vi "Write Error code.vi"(8 "error in (no error)":errorcluster, 10 "Error code":string, 11 "data_loader in":refnum<class "data_loader.lvclass">) -> (0 "error out":errorcluster, 3 "data_loader out":refnum<class "data_loader.lvclass">)   [LabVIEW 2017, in "data_loader.lvclass"]
uses:
  data_loader.lvclass
  data_loader.lvclass/data_loader.ctl
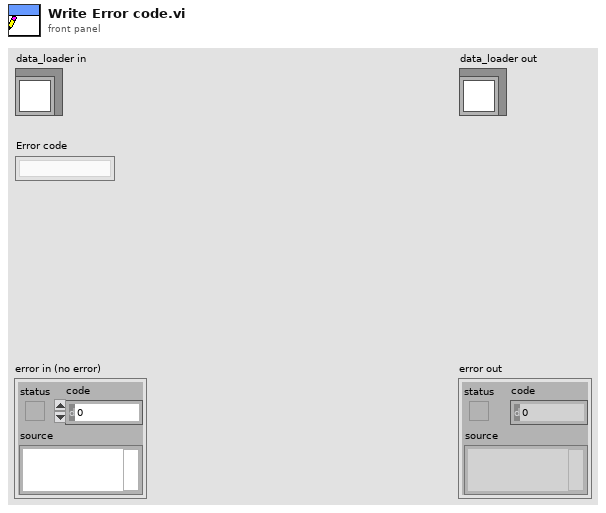
[diagram p1: front panel]
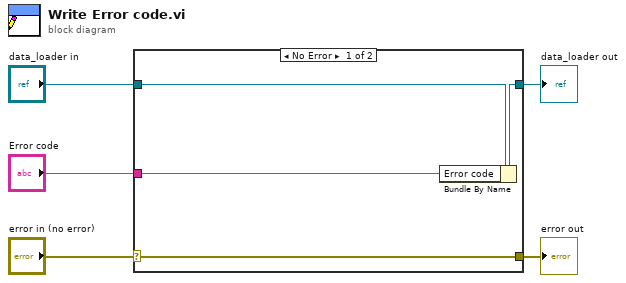
[diagram p0: block diagram]
diagram:
  n1 = case shown="No Error" "error in (no error)" {
    selector: "error in (no error)" -> [w9 w10]
    tunnel: [w9 w10] -> w4
    tunnel: [w7 w11] -> w2
    tunnel: "data_loader in" -> [w8 w11]
    tunnel: "Error code" -> [w6 _]
    frame No Error {
      n2 = Bundle By Name(cluster=w8, "Error code"=w6) -> (w7:refnum<class "data_loader.lvclass">)
    }
    frame Error {
    }
  }
  "error out" <- w4
  "data_loader out" <- w2
